vi "Build_Query_String.vi"(10 "Query parameters":cluster{"key":string, "value":string}[](array[cluster])) -> (2 "Query encoded string":string)   [LabVIEW 2019, in "ByteREST.lvlib" / "RESTBase.lvclass"]
uses:
  RESTBase.lvclass
  <vilib>/wsapi/NI_WebServices.lvlib
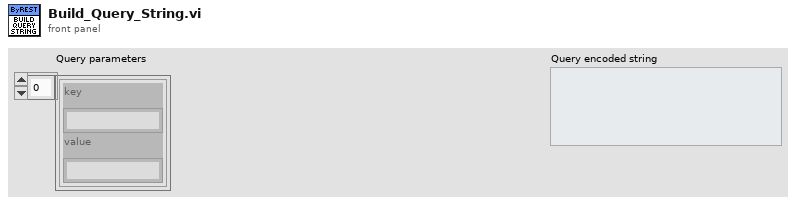
[diagram p1: front panel]
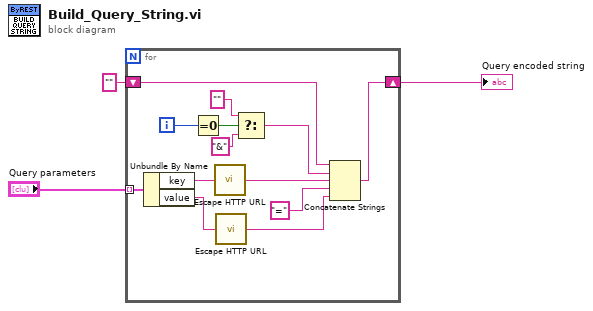
[diagram p0: block diagram]
diagram:
  n1 = for {
    tunnel: "Query parameters" -> [w16] mode=indexing
    shift-right: [w8] -> w1
    shift-left: "" -> [w9]
    i -> [w14]
    n2 = Unbundle By Name(w16) -> ("key"=w7:string, "value"=w5:string)
    n3 = Equal To 0?(x=w14) -> (x = 0?=w13:bool)
    n4 = call <vilib>:"Escape HTTP URL.vi"("unescaped string in"=w7) -> ("escaped string out"=w6:string)
    n5 = call <vilib>:"Escape HTTP URL.vi"("unescaped string in"=w5) -> ("escaped string out"=w4:string)
    n6 = Select(t="", s=w13, f="&") -> (s? t:f=w12:string)
    n7 = Concatenate Strings(w9, w12, w6, "=" ("string"), w4) -> (w8:string)
  }
  "Query encoded string" <- w1
